vi "TB-Init Stimulus.vi"(0 "Exposure parameters":T25={"Low cutoff (kHz)"=0.0, "High cutoff (kHz)"=0.0, "Duration (min)"=0.0, "dB SPL"=0.0, "Waveform"=enum."OFF", "WAVfile"=path "", "refWav"=path "", "use mic correction"=FALSE, "micCorrFile"=path "", "Pistonphone Level (dB SPL)"=0.0, "Sampling rate (Hz)"=0.0, "Buffer length (s)"=0.0, "Stream mic"=FALSE, "Fine adjust"={"Max"=0.0, "Min"=0.0}, "Mic gain"=0.0, "atten"=0.0, "resol (Hz)"=0.0, "navgs"=0, "Allow Slack"=FALSE, "max starts"=0, "Freq (kHz)"=8.0, "Tma (s)"=0.0, "Streamed"=[], "Drive"=""}, 7 "Sampling rate (Hz)":dbl, 9 "Npts":i32, 11 "error in (no error)":errorcluster, 13 "Exposure":bool) -> (4 "StimChan":T24(xcontrol), 6 "stimulus state":T1, 15 "error out":errorcluster)   [LabVIEW 2020]
uses:
  Typedefs/TB-Parameters.ctl
  epl-vi-lib/Signal Synthesis VIs/Controls/Waveform XCtl/Waveform Enum.ctl
  epl-vi-lib/Signal Synthesis VIs/Controls/Stimulus Channel XCtl/Stimulus Channel.xctl
  Typedefs/TB-Stimulus State.ctl
  <vilib>/sound2/lvsound2.llb/Sound File Refnum.ctl
  epl-vi-lib/Signal Synthesis VIs/Controls/Level XCtl/Level Units.ctl
  <vilib>/sound2/lvsound2.llb/Sound File Info (path).vi
  <vilib>/sound2/lvsound2.llb/Sound File Read Open.vi
  epl-vi-lib/Signal Synthesis VIs/Top Level VIs/Stimulus-Initialize.vi
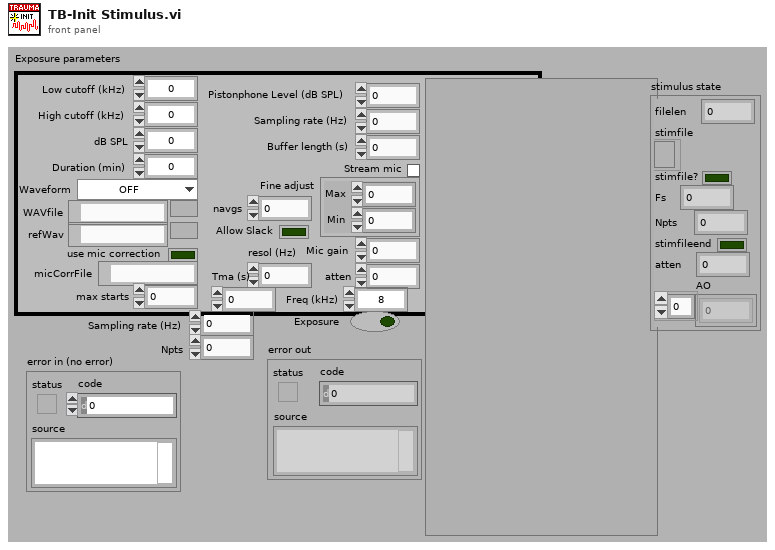
[diagram p1: front panel]
types:
  T1 = typedef "TB-Stimulus State.ctl" = cluster{"filelen":i32, "stimfile":T2, "stimfile?":bool, "Fs":dbl, "Npts":i32, "stimfileend":bool, "atten":dbl, "AO":i32[]}
  T2 = typedef "Sound File Refnum.ctl" = refnum<file>
  T3 = typedef "Waveform XCtl.xctl/Waveform Data.ctl" = cluster{"Type":T4, "Tone":T5, "Pulse Train":T6, "Noise":T9, "File":T10, "FMSweep":T11, "Chirp Train":T12, "Complex Tone":cluster{"Params":T14, "Data":T16}, "Moving Ripple":T17}
  T4 = typedef "Waveform Enum.ctl" = enum16{"OFF", "Tone", "Noise", "Pulse Train", "File", "FM Sweep", "Chirp Train", "Complex Tone", "FM Tone", "Moving Ripple"}
  T5 = typedef "Tone Params.ctl" = cluster{"Frequency (kHz)":dbl, "Last Freq":dbl, "Last Phase":dbl}
  T6 = typedef "Pulse Train Params.ctl" = cluster{"Pulse width (us)":dbl, "Pulse rate (Hz)":dbl, "Gap (ms)":dbl, "Polarity":T7, "PT State":T8, "Asynch":bool}
  T7 = typedef "Pulse Polarity.ctl" = enum16{"POS", "NEG", "POS-NEG", "NEG-POS"}
  T8 = typedef "PT-Continuous State.ctl" = cluster{"Template":dbl[], "Nperiod":i32, "Index":i32, "Pulse Rate (Hz)":dbl, "Phase (cycles)":dbl, "Noff":i32}
  T9 = typedef "Noise Params.ctl" = cluster{"InvFilt":bool, "Noise":dbl[], "CurPt":i32, "Aweight":bool, "Seed":i32, "afile":path}
  T10 = typedef "StimFile-Params.ctl" = cluster{"Filename":path, "Signal":dbl[], "Channel":i32, "stream":bool, "offset":i32, "nreps":i32, "loops":i32, "Randomize":bool, "order":i32[], "Seed":i32, "Tokens":i32}
  T11 = typedef "FM Sweep Params.ctl" = cluster{"Rate (oct/s)":dbl, "Fmin (Hz)":dbl, "Fmax (Hz)":dbl, "Ramp (ms)":dbl, "Linear":bool}
  T12 = typedef "Chirp Train.ctl" = cluster{"Params":T13, "Data":cluster{"WF":dbl[]}}
  T13 = typedef "Chirp Train Params.ctl" = cluster{"Fmin (kHz)":dbl, "Fmax (kHz)":dbl, "Compensate":bool, "Duration (ms)":dbl}
  T14 = typedef "CT-Params.ctl" = cluster{"F0 (Hz)":dbl, "Band":cluster{"Flow (Hz)":dbl, "Fhigh (Hz)":dbl}, "Phase":T15, "Min F0 (Hz)":dbl, "Max F0 (Hz)":dbl, "ContinRandPhase":bool, "Max peak factor":dbl, "Max mod depth":dbl, "MinHarmNum":i32, "MaxHarmNum":i32, "Level Mode":enum16{"per component", "overall rms"}, "% jitter":dbl}
  T15 = typedef "CT-Phase Enum.ctl" = enum16{"Cosine", "Random", "Alternating"}
  T16 = typedef "CT-Runtime Data.ctl" = cluster{"Ncomp":i32, "MinHarm":i32, "Phase":dbl[], "Amplitude":dbl[], "Npts/frame":i32, "Last F0":dbl, "Fmin":dbl, "Fmax":dbl, "Lslope":dbl, "randphase":bool, "overall rms":bool, "fmult":dbl[], "jittered":bool}
  T17 = typedef "Moving Ripple.ctl" = cluster{"Params":T18, "Data":T19}
  T18 = typedef "Moving Ripple.Params.ctl" = cluster{"Fmin":dbl, "Fmax":dbl, "Density":dbl, "Velocity":dbl, "Depth":dbl, "Phase":dbl, "Comp/oct":i32}
  T19 = typedef "Moving Ripple.Data.ctl" = cluster{"Freq":dbl[], "A":dbl[], "phase":dbl[], "Phase":dbl}
  T20 = typedef "Filter XCtl.xctl/Filter Data.ctl" = cluster{"CF (kHz)":dbl, "BW (kHz)":dbl, "IIR Filter Cluster":cluster{"filter structure":enum32{"IIR 2nd Order", "IIR 4th Order"}, "Reverse Coefficients":dbl[], "Forward Coefficients":dbl[]}, "Final Filter State":dbl[], "Scale Factor":dbl, "Final Filter State 2":dbl[], "Quadrature":bool, "Type":enum16{"Lowpass", "Highpass", "Bandpass", "Bandstop", "OFF"}}
  T21 = typedef "Gate Control.xctl/Gate Data.ctl" = cluster{"Active":bool, "Delay (ms)":dbl, "Width (ms)":dbl, "Ramp (ms)":dbl}
  T22 = typedef "Level XCtl.xctl/Level Data.ctl" = cluster{"Level":dbl, "Units":T23, "Max":dbl, "Multiplier":dbl, "Cal File":path, "Cal":cluster{"Freq (Hz)":dbl[], "Mag (dB SPL)":dbl[], "Phase (deg)":dbl[]}}
  T23 = typedef "Level Units.ctl" = enum16{"dB atten", "dB SPL", "dB re 1 Vrms", "dB V/Hz½", "mW", "dB HL", "Volts", "dB mW"}
  T24 = cluster{"Waveform":T3, "Filter":T20, "Gate":T21, "Level":T22}
  T25 = typedef "TB-Parameters.ctl" = cluster{"Low cutoff (kHz)":dbl, "High cutoff (kHz)":dbl, "Duration (min)":dbl, "dB SPL":dbl, "Waveform":T4, "WAVfile":path, "refWav":path, "use mic correction":bool, "micCorrFile":path, "Pistonphone Level (dB SPL)":dbl, "Sampling rate (Hz)":dbl, "Buffer length (s)":dbl, "Stream mic":bool, "Fine adjust":cluster{"Max":dbl, "Min":dbl}, "Mic gain":dbl, "atten":dbl, "resol (Hz)":dbl, "navgs":i32, "Allow Slack":bool, "max starts":i32, "Freq (kHz)":dbl, "Tma (s)":dbl, "Streamed":cluster{"Num":i32, "Name":string}[], "Drive":string}
  T26 = enum16{"Lowpass", "Highpass", "Bandpass", "Bandstop", "OFF"}
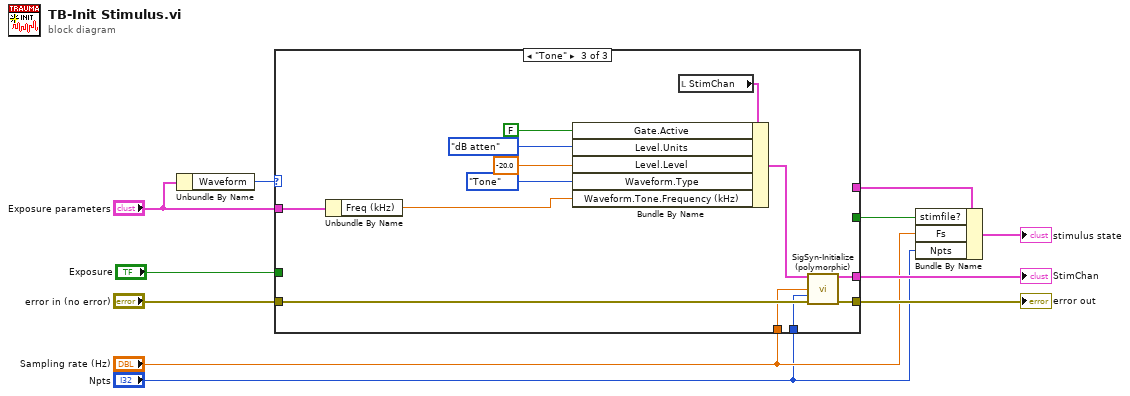
[diagram p0: block diagram]
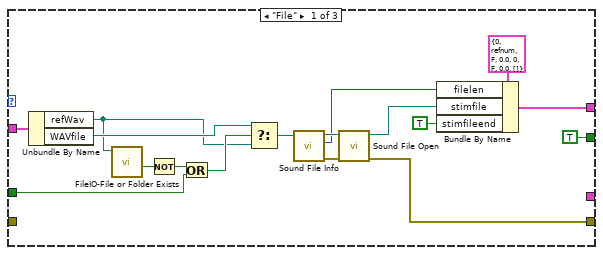
[diagram p2: hidden frame]
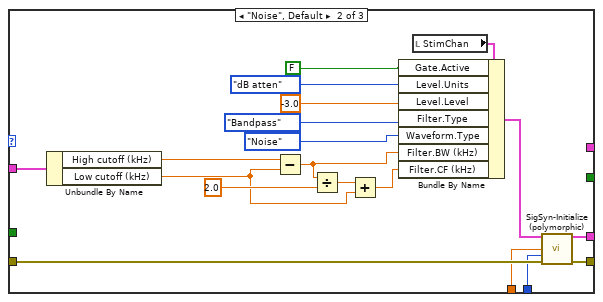
[diagram p3: hidden frame]
diagram:
  n1 = Unbundle By Name("Exposure parameters") -> ("Waveform"=w7:T4)
  n2 = case shown="\"Tone\"" w7 {
    tunnel: "error in (no error)" -> [_ w34 w54]
    tunnel: [w27 w33 w53] -> w10
    tunnel: "Sampling rate (Hz)" -> [_ w32 w52]
    tunnel: [_ w30 w50] -> w9
    tunnel: "Exposure parameters" -> [w28 w29 w49]
    tunnel: [w23 _ _] -> w6
    tunnel: "Npts" -> [_ w31 w51]
    tunnel: [TRUE _ _] -> w4
    tunnel: "Exposure" -> [w19 _ _]
    frame "File" {
      n3 = Unbundle By Name(w28) -> ("refWav"=w16:path, "WAVfile"=w17:path)
      n4 = call "FileIO-File or Folder Exists.vi"("path"=w16) -> ("Exists?"=w21:bool)  [unwired: 7 in, 3 out]
      n5 = Not(x=w21) -> (.not. x?=w20:bool)
      n6 = Or(x=w20, y=w19) -> (x .or. y?=w18:bool)
      n7 = Select(t=w17, s=w18, f=w16) -> (s? t:f=w15:path)
      n8 = call-poly <vilib>:"Sound File Info.vi"("path"=w15) -> ("error out"=w26:errorcluster, "total number of samples/ch"=w24:u32, "path out"=w25:path)  [unwired: 7 in, 1 out]
      n9 = call-poly <vilib>:"Sound File Open.vi"("error in (no error)"=w26, "path"=w25) -> ("error out"=w27:errorcluster, "sound file refnum"=w14:T2)  [unwired: 8 in]
      n10 = Bundle By Name(cluster=T1 {"filelen"=0, "stimfile"=refnum, "stimfile?"=FALSE, "Fs"=0.0, "Npts"=0, "stimfileend"=FALSE, "atten"=0.0, "AO"=[]} ("state"), "filelen"=w24, "stimfile"=w14, "stimfileend"=TRUE) -> (w23:T1)
    }
    frame "Noise", Default {
      n11 = Unbundle By Name(w29) -> ("High cutoff (kHz)"=w41:dbl, "Low cutoff (kHz)"=w37:dbl)
      n12 = Subtract(x=w41, y=w37) -> (x-y=w40:dbl)
      n13 = Divide(x=w40, y=2.0) -> (x/y=w38:dbl)
      n14 = Add(x=w38, y=w37) -> (x+y=w36:dbl)
      n15 = local read "StimChan"() -> (w47:T24)
      n16 = Bundle By Name(cluster=w47, "Gate.Active"=FALSE, "Level.Units"=Level_Units."dB atten" ("Level.Mode"), "Level.Level"=-3.0, "Filter.Type"=T26."Bandpass", "Waveform.Type"=Waveform_Enum."Noise", "Filter.BW (kHz)"=w40, "Filter.CF (kHz)"=w36) -> (w35:T24)
      n17 = call-poly "SigSyn-Initialize (polymorphic).vi"("Stimulus Channel"=w35, "Sampling rate (Hz)"=w32, "Npts"=w31, "error in (no error)"=w34) -> ("Stimulus Channel out"=w30:T24, "error out"=w33:errorcluster)  [unwired: 9 in, 1 out]
    }
    frame "Tone" {
      n18 = Unbundle By Name(w49) -> ("Freq (kHz)"=w48:dbl)
      n19 = local read "StimChan"() -> (w60:T24)
      n20 = Bundle By Name(cluster=w60, "Gate.Active"=FALSE, "Level.Units"=Level_Units."dB atten" ("Level.Mode"), "Level.Level"=-20.0, "Waveform.Type"=Waveform_Enum."Tone", "Waveform.Tone.Frequency (kHz)"=w48) -> (w55:T24)
      n21 = call-poly "SigSyn-Initialize (polymorphic).vi"("Stimulus Channel"=w55, "Sampling rate (Hz)"=w52, "Npts"=w51, "error in (no error)"=w54) -> ("Stimulus Channel out"=w50:T24, "error out"=w53:errorcluster)  [unwired: 9 in, 1 out]
    }
  }
  "error out" <- w10
  "StimChan" <- w9
  n22 = Bundle By Name(cluster=w6, "stimfile?"=w4, "Fs"="Sampling rate (Hz)", "Npts"="Npts") -> (→"stimulus state":T1)
